vi "Blinking LED Multiple Loop.vi"() -> ()   [LabVIEW 2014]
uses:
  WiringPI GPIO TypeDef.ctl
  libgpio_exp02.so
panel:
  out "Status 4":bool
  out "Status 3":bool
  out "Status 2":bool
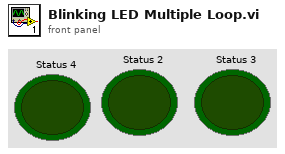
[diagram p1: front panel]
types:
  T1 = typedef "WiringPI GPIO TypeDef.ctl" = u8
  T2 = enum8{"INPUT", "OUTPUT", "PWM_OUTPUT", "GPIO_CLOCK", "SOFT_PWM_OUTPUT", "SOFT_TONE_OUTPUT", "PWM_TONE_OUTPUT"}
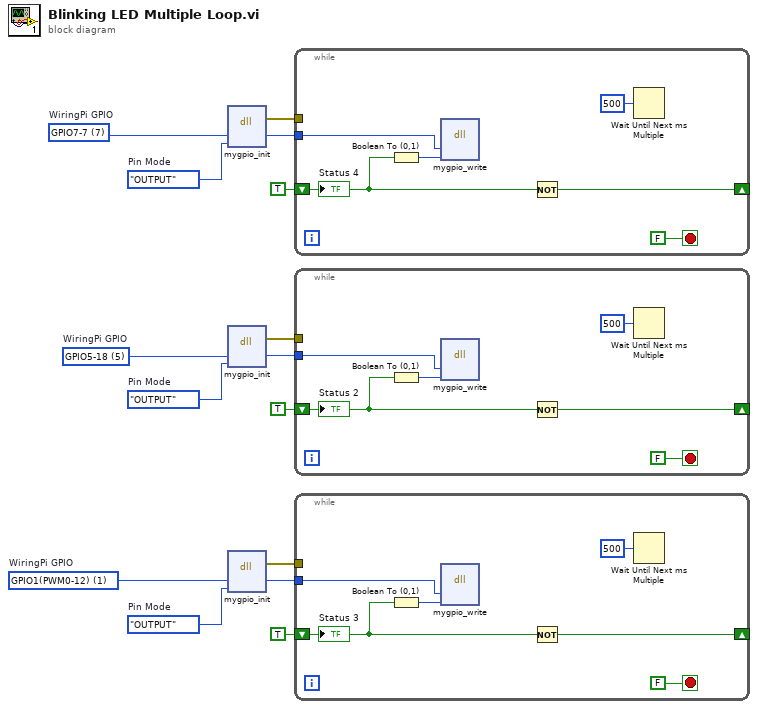
[diagram p0: block diagram]
diagram:
  w3 = T1 1 items=["SDA(I2C)-3"=8, "SCL(I2C)-5"=9, "MOSI(SPI)-19"=12, "MISO(SPI)-21"=13, "SCLK(SPI)-23"=14, "GPIO4-16"=4, "GPIO5-18"=5, "GPIO6-22"=6, "GPIO7-7"=7, "GPIO21-29"=21, "GPIO22-31"=22, "GPIO25-37"=25, "GPIO27-36"=27, "GPIO26(PWM0)-32"=26, "GPIO1(PWM0-12)"=1, "GPIO23(PWM1)-14"=23, "GPIO24(PWM1)-35"=24, "TXD(UART)-8"=15, "RXD(UART)-10"=16, "GPIO10(CE0-SPI)-24"=10, "GPPI11(CE1)-SPI)-26"=11, "GPIO28(PCM_DIN)36"=28, "GPIO29(PCM_DOUT)40"=29]  # WiringPi GPIO
  w2 = T1 5 items=["SDA(I2C)-3"=8, "SCL(I2C)-5"=9, "MOSI(SPI)-19"=12, "MISO(SPI)-21"=13, "SCLK(SPI)-23"=14, "GPIO4-16"=4, "GPIO5-18"=5, "GPIO6-22"=6, "GPIO7-7"=7, "GPIO21-29"=21, "GPIO22-31"=22, "GPIO25-37"=25, "GPIO27-36"=27, "GPIO26(PWM0)-32"=26, "GPIO1(PWM0-12)"=1, "GPIO23(PWM1)-14"=23, "GPIO24(PWM1)-35"=24, "TXD(UART)-8"=15, "RXD(UART)-10"=16, "GPIO10(CE0-SPI)-24"=10, "GPPI11(CE1)-SPI)-26"=11, "GPIO28(PCM_DIN)36"=28, "GPIO29(PCM_DOUT)40"=29]  # WiringPi GPIO
  w1 = T1 7 items=["SDA(I2C)-3"=8, "SCL(I2C)-5"=9, "MOSI(SPI)-19"=12, "MISO(SPI)-21"=13, "SCLK(SPI)-23"=14, "GPIO4-16"=4, "GPIO5-18"=5, "GPIO6-22"=6, "GPIO7-7"=7, "GPIO21-29"=21, "GPIO22-31"=22, "GPIO25-37"=25, "GPIO27-36"=27, "GPIO26(PWM0)-32"=26, "GPIO1(PWM0-12)"=1, "GPIO23(PWM1)-14"=23, "GPIO24(PWM1)-35"=24, "TXD(UART)-8"=15, "RXD(UART)-10"=16, "GPIO10(CE0-SPI)-24"=10, "GPPI11(CE1)-SPI)-26"=11, "GPIO28(PCM_DIN)36"=28, "GPIO29(PCM_DOUT)40"=29]  # WiringPi GPIO
  w4 = T2."OUTPUT"  # Pin Mode
  w8 = T2."OUTPUT"  # Pin Mode
  w15 = T2."OUTPUT"  # Pin Mode
  n1 = dll-call lib="libgpio_exp02.so" fn="mygpio_init"("pin"=w1, "mode"=w4) -> (error out=w6:errorcluster, "pin"=w7:u8)  [unwired: 5 in, 1 out]
  n2 = dll-call lib="libgpio_exp02.so" fn="mygpio_init"("pin"=w2, "mode"=w15) -> (error out=w13:errorcluster, "pin"=w12:u8)  [unwired: 5 in, 1 out]
  n3 = dll-call lib="libgpio_exp02.so" fn="mygpio_init"("pin"=w3, "mode"=w8) -> (error out=w10:errorcluster, "pin"=w11:u8)  [unwired: 5 in, 1 out]
  n4 = while {
    tunnel: w6 -> [_]
    shift-right: [w17] -> _
    shift-left: TRUE -> [w20]
    tunnel: w7 -> [w16]
    stop <- FALSE stop-if-true
    n5 = Boolean To (0,1)(Boolean=w20) -> (0, 1=w21:i16)
    n6 = dll-call lib="libgpio_exp02.so" fn="mygpio_write"("pin"=w16, "state"=w21) -> ()  [unwired: 6 in, 2 out]
    n7 = Not(x=w20) -> (.not. x?=w17:bool)
    n8 = Wait Until Next ms Multiple(millisecond multiple=u32 500) -> ()  [unwired: 1 out]
    "Status 4" <- w20
  }
  n9 = while {
    tunnel: w13 -> [_]
    shift-right: [w23] -> _
    shift-left: TRUE -> [w26]
    tunnel: w12 -> [w22]
    stop <- FALSE stop-if-true
    n10 = Boolean To (0,1)(Boolean=w26) -> (0, 1=w27:i16)
    n11 = dll-call lib="libgpio_exp02.so" fn="mygpio_write"("pin"=w22, "state"=w27) -> ()  [unwired: 6 in, 2 out]
    n12 = Not(x=w26) -> (.not. x?=w23:bool)
    n13 = Wait Until Next ms Multiple(millisecond multiple=u32 500) -> ()  [unwired: 1 out]
    "Status 2" <- w26
  }
  n14 = while {
    tunnel: w10 -> [_]
    shift-right: [w29] -> _
    shift-left: TRUE -> [w32]
    tunnel: w11 -> [w28]
    stop <- FALSE stop-if-true
    n15 = Boolean To (0,1)(Boolean=w32) -> (0, 1=w33:i16)
    n16 = dll-call lib="libgpio_exp02.so" fn="mygpio_write"("pin"=w28, "state"=w33) -> ()  [unwired: 6 in, 2 out]
    n17 = Not(x=w32) -> (.not. x?=w29:bool)
    n18 = Wait Until Next ms Multiple(millisecond multiple=u32 500) -> ()  [unwired: 1 out]
    "Status 3" <- w32
  }
